vi "AH2500Monitor.VI"() -> ()   [LabVIEW 2019]
uses:
  Utility/Monitor Communication/AH2500/AH2500-Cluster.ctl
  Instrument_Setup.vi
  Global/Global Variables/Data_Display_global.vi
panel:
  in  "error in (no error)":errorcluster caption="Fehler (Eingang, kein Fehler)"
  in  "Stopp":bool
  out "AH2500-Cluster":T1
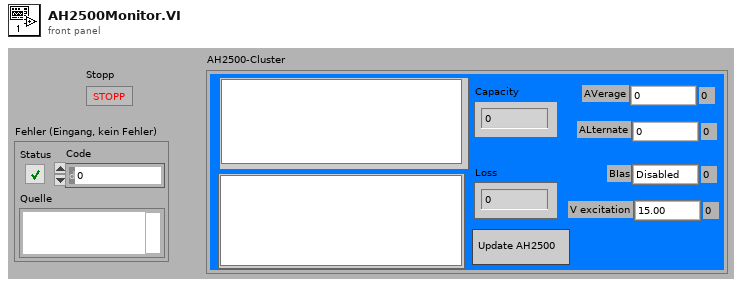
[diagram p1: front panel]
types:
  T1 = typedef "AH2500-Cluster.ctl" = cluster{"Capacity Graphic":dbl[][], "Loss Graphic":dbl[][], "Update AH2500":bool, "Capacity":dbl, "Loss":dbl, "AVerage":enum16{"0", "1", "2", "3", "4", "5", "6", "7", "8", "9", "10", "11", "12", "13", "14", "15"}, "ALternate":enum16{"0", "1", "2", "3", "4", "5", "6", "7"}, "BIas":enum16{"Disabled", "100 MOhm", "1 MOhm"}, "V excitation":enum16{"15.00", "7.50", "3.75", "3.00", "1.50", "0.750", "0.375", "0.250", "0.125", "0.100", "0.050", "0.030", "0.015", "0.010", "0.0050", "0.0030", "0.0015", "0.0010", "0.0005"}}
  T2 = cluster{"AVerage":dbl, "Alternate":dbl, "Bias":dbl, "V excitation":dbl}
  T3 = enum16{"0", "1", "2", "3", "4", "5", "6", "7", "8", "9", "10", "11", "12", "13", "14", "15"}
  T4 = enum16{"15.00", "7.50", "3.75", "3.00", "1.50", "0.750", "0.375", "0.250", "0.125", "0.100", "0.050", "0.030", "0.015", "0.010", "0.0050", "0.0030", "0.0015", "0.0010", "0.0005"}
  T5 = typedef "AH2500-Control.ctl" = cluster{"Update AH2500":bool}
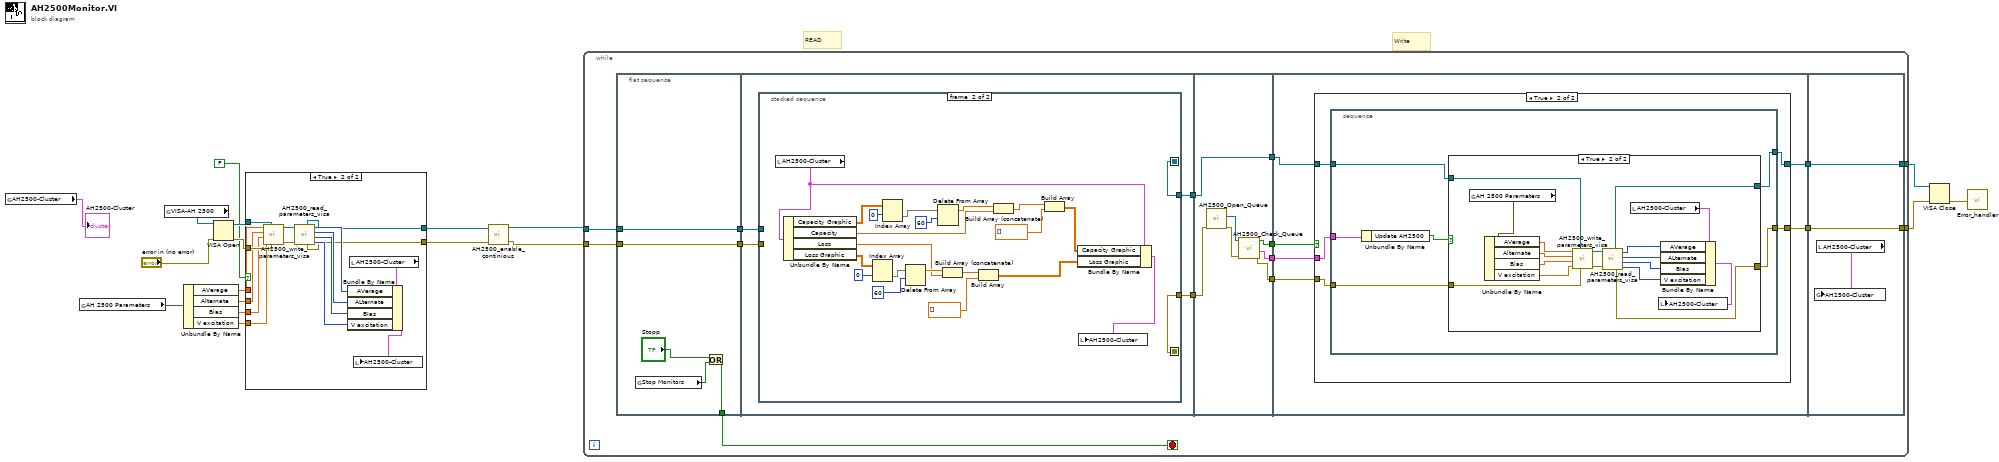
[diagram p0: block diagram]
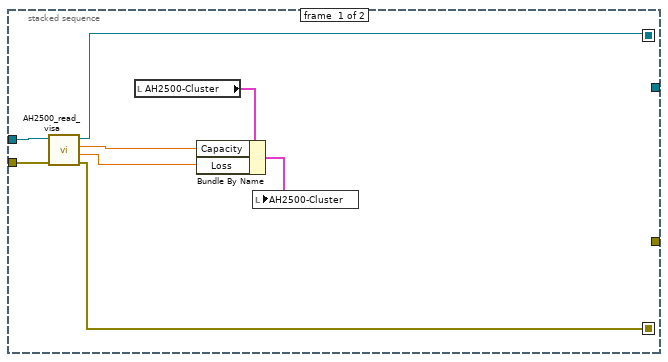
[diagram p3: hidden frame]
diagram:
  # "Write"
  # "READ"
  n1 = global read "Data_Display_global.vi" "AH2500-Cluster"() -> (→"AH2500-Cluster":T1)
  n2 = global read "Instrument_Setup.vi" "AH 2500 Parameters"() -> (w11:T2)
  n3 = global read "Instrument_Setup.vi" "VISA-AH 2500"() -> (w18:refnum<visa-resource-name>)
  n4 = Unbundle By Name(w11) -> ("AVerage"=w10:dbl, "Alternate"=w9:dbl, "Bias"=w8:dbl, "V excitation"=w7:dbl)
  n5 = VISA Open(error in (no error)="error in (no error)", VISA resource name=w18) -> (VISA resource name=w13:refnum<visa-resource-name>, error out=w12:errorcluster)  [unwired: 3 in]
  n6 = case shown="True" FALSE {
    tunnel: [w20 w22] -> w4
    tunnel: [w19 w21] -> w2
    tunnel: w13 -> [w20 w36]
    tunnel: w12 -> [w19 w35]
    tunnel: w10 -> [_ w34]
    tunnel: w9 -> [_ w33]
    tunnel: w8 -> [_ w32]
    tunnel: w7 -> [_ w31]
    frame False {
    }
    frame True {
      n7 = call "AH2500_write_parameters_visa.vi"("error in (no error)"=w35, "AH2500-Visa-address"=w36, "V excitation"=w31, "BIas"=w32, "ALternate"=w33, "AVerage"=w34) -> ("error out"=w29:errorcluster, "AH2500-Visa-adress-dub"=w30:refnum<visa-resource-name>)  [unwired: 2 in]
      n8 = call "AH2500_read_parameters_visa.vi"("VISA-AH2500"=w30, "error in (no error)"=w29) -> ("VISA-AH2500 dub"=w22:refnum<visa-resource-name>, "error out"=w21:errorcluster, "AVerage"=w26:T3, "ALternate"=w25:enum16{"0", "1", "2", "3", "4", "5", "6", "7"}, "BIas"=w24:enum16{"Disabled", "100 MOhm", "1 MOhm"}, "V excitation 2"=w23:T4)  [unwired: 2 in]
      n9 = local read "AH2500-Cluster"() -> (w28:T1)
      n10 = Bundle By Name(cluster=w28, "AVerage"=w26, "ALternate"=w25, "BIas"=w24, "V excitation"=w23) -> (w27:T1)
      n11 = local write "AH2500-Cluster"(w27) -> ()
    }
  }
  n12 = call "AH2500_enable_continious.vi"("error in (no error)"=w2, "AH2500-visa-address"=w4) -> ("error out"=w1:errorcluster, "AH2500-visa-address-dup"=w3:refnum<visa-resource-name>)  [unwired: 2 in]
  n13 = while {
    tunnel: w3 -> [w49]
    tunnel: w1 -> [w47]
    tunnel: [w40] -> w15
    tunnel: [w39] -> w16
    stop <- w51 stop-if-true
    n14 = flat-sequence {
      tunnel: [w54] -> w51
      tunnel: [w53] -> w50
      tunnel: w49 -> [w53]
      tunnel: [w52] -> w48
      tunnel: w47 -> [w52]
      tunnel: w50 -> [w60]
      tunnel: w48 -> [w59]
      tunnel: [w58] -> w46
      tunnel: [w57] -> w45
      tunnel: w46 -> [w91]
      tunnel: w45 -> [w97]
      tunnel: [w94] -> w44
      tunnel: [w93] -> w43
      tunnel: [w92] -> w42
      tunnel: [w91] -> w41
      tunnel: w44 -> [w103]
      tunnel: w43 -> [w102]
      tunnel: w42 -> [w101]
      tunnel: w41 -> [w100]
      tunnel: [w99] -> w38
      tunnel: [w98] -> w37
      tunnel: [w137] -> w39
      tunnel: [w138] -> w40
      tunnel: w38 -> [w138]
      tunnel: w37 -> [w137]
      frame #0 {
        n15 = global read "Data_Display_global.vi" "Stop Monitors"() -> (w55:bool)
        n16 = Or(x="Stopp", y=w55) -> (x .or. y?=w54:bool)
      }
      frame #1 {
        n17 = stacked-sequence {
          seq-local: [w61 _] -> [_ w70]
          seq-local: [w62 _] -> [_ w69]
          tunnel: w60 -> [w63 _]
          tunnel: w59 -> [w68 _]
          tunnel: [_ w70] -> w58
          tunnel: [_ w69] -> w57
          frame #0 {
            n18 = call "AH2500_read_visa.vi"("error in (no error)"=w68, "VISA-AH2500A-address"=w63) -> ("error out"=w62:errorcluster, "loss"=w64:dbl, "capacitance"=w65:dbl, "VISA-AH2500A-address dub"=w61:refnum<visa-resource-name>)  [unwired: 2 in]
            n19 = local read "AH2500-Cluster"() -> (w67:T1)
            n20 = Bundle By Name(cluster=w67, "Capacity"=w65, "Loss"=w64) -> (w66:T1)
            n21 = local write "AH2500-Cluster"(w66) -> ()
          }
          frame #1 {
            n22 = local read "AH2500-Cluster"() -> (w90:T1)
            n23 = Unbundle By Name(w90) -> ("Capacity Graphic"=w84:dbl[][], "Capacity"=w79:dbl, "Loss"=w77:dbl, "Loss Graphic"=w83:dbl[][])
            n24 = Index Array(array=w83, index (row)=0) -> (element=w86:dbl[])  [unwired: 1 in]
            n25 = Index Array(array=w84, index (row)=0) -> (element=w85:dbl[])  [unwired: 1 in]
            n26 = Delete From Array(array=w86, length=60) -> (array with subset deleted=w78:dbl[])  [unwired: 1 in, 1 out]
            n27 = Delete From Array(array=w85, length=60) -> (array with subset deleted=w80:dbl[])  [unwired: 1 in, 1 out]
            n28 = Build Array (concatenate)(w78, w77) -> (w73:dbl[])
            n29 = Build Array(w73, dbl[] []) -> (w71:dbl[][])
            n30 = Build Array (concatenate)(w80, w79) -> (w76:dbl[])
            n31 = Build Array(w76, dbl[] []) -> (w74:dbl[][])
            n32 = Bundle By Name(cluster=w90, "Capacity Graphic"=w74, "Loss Graphic"=w71) -> (w89:T1)
            n33 = local write "AH2500-Cluster"(w89) -> ()
          }
        }
      }
      frame #2 {
        n34 = call "AH2500_Open_Queue.vi"("error in (no error)"=w97) -> ("error out"=w96:errorcluster, "queue out"=w95:refnum<queue>)  [unwired: 9 in]
        n35 = call "AH2500_Check_Queue.vi"("error in (no error)"=w96, "Queue"=w95) -> ("error out"=w92:errorcluster, "AH2500-Control"=w93:T5, "New Entries?"=w94:bool)  [unwired: 6 in]
      }
      frame #3 {
        n36 = case shown="True" w103 {
          tunnel: w102 -> [_ w110]
          tunnel: w101 -> [w105 w109]
          tunnel: w100 -> [w104 w108]
          tunnel: [w105 w107] -> w99
          tunnel: [w104 w106] -> w98
          frame False {
          }
          frame True {
            n37 = stacked-sequence {
              tunnel: w110 -> [w116]
              tunnel: w109 -> [w114]
              tunnel: w108 -> [w113]
              tunnel: [w112] -> w107
              tunnel: [w111] -> w106
              frame #0 {
                n38 = Unbundle By Name(w116) -> ("Update AH2500"=w115:bool)
                n39 = case shown="True" w115 {
                  tunnel: w114 -> [w118 w130]
                  tunnel: [w118 w127] -> w112
                  tunnel: w113 -> [w117 w129]
                  tunnel: [w117 w125] -> w111
                  frame False {
                  }
                  frame True {
                    n40 = global read "Instrument_Setup.vi" "AH 2500 Parameters"() -> (w135:T2)
                    n41 = Unbundle By Name(w135) -> ("AVerage"=w134:dbl, "Alternate"=w133:dbl, "Bias"=w132:dbl, "V excitation"=w131:dbl)
                    n42 = call "AH2500_write_parameters_visa.vi"("error in (no error)"=w130, "AH2500-Visa-address"=w129, "V excitation"=w131, "BIas"=w132, "ALternate"=w133, "AVerage"=w134) -> ("error out"=w128:errorcluster, "AH2500-Visa-adress-dub"=w126:refnum<visa-resource-name>)  [unwired: 2 in]
                    n43 = call "AH2500_read_parameters_visa.vi"("VISA-AH2500"=w126, "error in (no error)"=w128) -> ("VISA-AH2500 dub"=w125:refnum<visa-resource-name>, "error out"=w127:errorcluster, "AVerage"=w122:T3, "ALternate"=w121:enum16{"0", "1", "2", "3", "4", "5", "6", "7"}, "BIas"=w120:enum16{"Disabled", "100 MOhm", "1 MOhm"}, "V excitation 2"=w119:T4)  [unwired: 2 in]
                    n44 = local read "AH2500-Cluster"() -> (w124:T1)
                    n45 = Bundle By Name(cluster=w124, "AVerage"=w122, "ALternate"=w121, "BIas"=w120, "V excitation"=w119) -> (w123:T1)
                    n46 = local write "AH2500-Cluster"(w123) -> ()
                  }
                }
              }
            }
          }
        }
      }
      frame #4 {
        n47 = local read "AH2500-Cluster"() -> (w136:T1)
        n48 = global write "Data_Display_global.vi" "AH2500-Cluster"(w136) -> ()
      }
    }
  }
  n49 = VISA Close(VISA resource name=w16, error in (no error)=w15) -> (error out=w6:errorcluster)
  n50 = call "Error_handler.vi"("error constant"=w6) -> ()
